vi "HandleObservationSync_002.vi"(8 "error in (no error)":errorcluster, 11 "S4GUI in":refnum<class "S4GUI.lvclass">) -> (0 "error out":errorcluster, 3 "S4GUI out":refnum<class "S4GUI.lvclass">)   [LabVIEW 2018, in "S4GUI.lvclass"] (continued)
            tunnel: [w1984 w1997] -> w1912
            tunnel: [w1983 w1996] -> w1911
            tunnel: [0 ("State") w1986] -> w1887
            frame False {
            }
            frame True {
              n759 = call-dynamic "Read Channel.vi"("error in (no error)"=w1999, "Acquisition in"=w2000) -> ("error out"=w1995:errorcluster, "Channel.lvclass"=w1994:refnum<class "Channel.lvclass">, "Acquisition out"=w1998:refnum<class "Acquisition.lvclass">)  [unwired: 7 in]
              n760 = call-dynamic "Read State Machine.vi"("error in (no error)"=w1995, "Device in"=w1994) -> ("error out"=w1988:errorcluster, "State Machine.lvclass"=w1990:refnum<class "State Machine.lvclass">, "Device out"=w1992:refnum<class "Channel.lvclass">)  [unwired: 7 in]
              n761 = call-dynamic "Read State.vi"("error in (no error)"=w1988, "State Machine in"=w1990) -> ("error out"=w1987:errorcluster, "State"=w1986:i32, "State Machine out"=w1989:refnum<class "State Machine.lvclass">)  [unwired: 7 in]
              n762 = call-dynamic "Write State Machine.vi"("error in (no error)"=w1987, "State Machine.lvclass"=w1989, "Device in"=w1992) -> ("error out"=w1991:errorcluster, "Device out"=w1993:refnum<class "Channel.lvclass">)  [unwired: 7 in]
              n763 = call-dynamic "Write Channel.vi"("error in (no error)"=w1991, "Channel.lvclass"=w1993, "Acquisition in"=w1998) -> ("error out"=w1996:errorcluster, "Acquisition out"=w1997:refnum<class "Acquisition.lvclass">)  [unwired: 7 in]
            }
          }
          n764 = call-dynamic "Write AcquisitionC.vi"("error in (no error)"=w1911, "Acquisition.lvclass"=w1912, "S4ACS_GUI in"=w1941) -> ("error out"=w1935:errorcluster, "S4ACS_GUI out"=w1934:refnum<class "S4GUI.lvclass">)  [unwired: 7 in]
          n765 = call-dynamic "Read AcquisitionD.vi"("error in (no error)"=w1935, "S4ACS_GUI in"=w1934) -> ("error out"=w1908:errorcluster, "Acquisition.lvclass"=w1910:refnum<class "Acquisition.lvclass">, "S4ACS_GUI out"=w1940:refnum<class "S4GUI.lvclass">)  [unwired: 7 in]
          n766 = call "Read connection.vi"("error in (no error)"=w1908, "Server in"=w1910) -> ("error out"=w1907:errorcluster, "connection"=w1906:bool, "Server out"=w1909:refnum<class "Acquisition.lvclass">)  [unwired: 7 in]
          n767 = case shown="True" w1906 {
            tunnel: w1909 -> [w1966 w1982]
            tunnel: w1907 -> [w1965 w1981]
            tunnel: [w1966 w1979] -> w1905
            tunnel: [w1965 w1978] -> w1904
            tunnel: [0 ("State") w1968] -> w1886
            frame False {
            }
            frame True {
              n768 = call-dynamic "Read Channel.vi"("error in (no error)"=w1981, "Acquisition in"=w1982) -> ("error out"=w1977:errorcluster, "Channel.lvclass"=w1976:refnum<class "Channel.lvclass">, "Acquisition out"=w1980:refnum<class "Acquisition.lvclass">)  [unwired: 7 in]
              n769 = call-dynamic "Read State Machine.vi"("error in (no error)"=w1977, "Device in"=w1976) -> ("error out"=w1970:errorcluster, "State Machine.lvclass"=w1972:refnum<class "State Machine.lvclass">, "Device out"=w1974:refnum<class "Channel.lvclass">)  [unwired: 7 in]
              n770 = call-dynamic "Read State.vi"("error in (no error)"=w1970, "State Machine in"=w1972) -> ("error out"=w1969:errorcluster, "State"=w1968:i32, "State Machine out"=w1971:refnum<class "State Machine.lvclass">)  [unwired: 7 in]
              n771 = call-dynamic "Write State Machine.vi"("error in (no error)"=w1969, "State Machine.lvclass"=w1971, "Device in"=w1974) -> ("error out"=w1973:errorcluster, "Device out"=w1975:refnum<class "Channel.lvclass">)  [unwired: 7 in]
              n772 = call-dynamic "Write Channel.vi"("error in (no error)"=w1973, "Channel.lvclass"=w1975, "Acquisition in"=w1980) -> ("error out"=w1978:errorcluster, "Acquisition out"=w1979:refnum<class "Acquisition.lvclass">)  [unwired: 7 in]
            }
          }
          n773 = call-dynamic "Write AcquisitionD.vi"("error in (no error)"=w1904, "Acquisition.lvclass"=w1905, "S4ACS_GUI in"=w1940) -> ("error out"=w1933:errorcluster, "S4ACS_GUI out"=w1898:refnum<class "S4GUI.lvclass">)  [unwired: 7 in]
          n774 = Equal?(x=w1890, y=w1889) -> (x = y?=w1894:bool)
          n775 = Equal?(x=w1899, y=w1889) -> (x = y?=w1903:bool)
          n776 = Equal?(x=w1890, y=w1888) -> (x = y?=w1893:bool)
          n777 = Equal?(x=w1899, y=w1888) -> (x = y?=w1902:bool)
          n778 = Equal?(x=w1890, y=w1887) -> (x = y?=w1892:bool)
          n779 = Equal?(x=w1899, y=w1887) -> (x = y?=w1901:bool)
          n780 = Equal?(x=w1890, y=w1886) -> (x = y?=w1891:bool)
          n781 = Equal?(x=w1899, y=w1886) -> (x = y?=w1900:bool)
          n782 = Compound Arithmetic op=ADD(w1889, w1888, w1887, w1886) -> (w1897:i32)
          n783 = Compound Arithmetic op=OR(w1894, w1893, w1892, w1891) -> (w1884:bool)
          n784 = Compound Arithmetic op=OR(w1903, w1902, w1901, w1900) -> (w1885:bool)
          n785 = Build Array(w1885, w1884) -> (w1883:bool[])
          n786 = Boolean Array To Number(Boolean array=w1883) -> (number=w1882:u32)
          n787 = case shown="0, Default" w1882 {
            tunnel: w1898 -> [w1948 w1956 w1960 w1964]
            tunnel: [w1947 w1955 w1959 w1963] -> w1895
            tunnel: w1897 -> [w1952 _ _ _]
            tunnel: w1896 -> [w1949 _ _ _]
            frame 0, Default {
              n788 = Equal To 0?(x=w1952) -> (x = 0?=w1951:bool)
              n789 = Select(t=u32 360, s=w1951, f=w1949) -> (s? t:f=w1946:u32)
              n790 = Bundle By Name(cluster=w1948, "Obs_state"=w1946) -> (w1947:refnum<class "S4GUI.lvclass">)
            }
            frame 1 {
              n791 = Bundle By Name(cluster=w1956, "Obs_state"=u32 1, "Error Msg"="ERROR: Some channel initialization failed. S4GUI:HandleObservationSync.vi state 272.") -> (w1955:refnum<class "S4GUI.lvclass">)
            }
            frame 2 {
              n792 = Bundle By Name(cluster=w1960, "Obs_state"=u32 1, "Error Msg"="ERROR: Some channel with invalid Exposition Time. S4GUI:HandleObservationSync.vi state 272.") -> (w1959:refnum<class "S4GUI.lvclass">)
            }
            frame 3 {
              n793 = Bundle By Name(cluster=w1964, "Obs_state"=u32 1, "Error Msg"="ERROR: Invalid configuration in the channels. S4GUI:HandleObservationSync.vi state 272.") -> (w1963:refnum<class "S4GUI.lvclass">)
            }
          }
        }
        frame 299 {
          # "Verifcando iniciação dos CICLO:"
          # "T= todos os canais ativos estão zerados."
          # "Exemplo de erro em \"Cycles_done\":\nchA; cycles_done=0; CCD_STATUS=ACTIVE;                                           Seqs_done=15;\nchA; cycles_done=0; CCD_STATUS=IDLE;                                                Seqs_done=16;   =>mudança de seq. com mesmo ciclo\nchA; cycles_done=1; CCD_STATUS=WAITING_EXPOSE_COMMAND; Seqs_done=0;\n\nchB; cycles_done=0; CCD_STATUS=ACTIVE;                                           Seqs_done=15;\nchB; cycles_done=1; CCD_STATUS=WAITING_EXPOSE_COMMAND; Seqs_done=0;     => mudança de seq com novo ciclo"
          # "T=canais receberam STOP"
          # "T= Todos os canais ativos no mesmo ciclo;\nF= Canais em ciclo diferente."
          # "Todos os CYCLES_DONE \nestão zerados?\nSe sim, vai para 327."
          # "Exemplo:\nSET #CYCLES 3\nSET #SEQ 4\ntotal de sequencias: 3 x 4 = 12\n\nseq.        CYCLES_DONE           SEQS_DONE\n1a.                     0                                 0\n2a.                     0                                 1 \n3a.                     0                                 2 \n4a.                     0                                 3 \n                          1                                 4\n5a.                     1                                 0 \n6a.                     1                                 1 \n7a.                     1                                 2 \n8a.                     1                                 3 \n                          2                                 4\n9a.                     2                                 0 \n10a.                   2                                 1 \n11a.                   2                                 2 \n12a.                   2                                 3 \n\nfim                    3                                 4"
          n794 = call-dynamic "Read AcquisitionA.vi"("error in (no error)"=w2089, "S4ACS_GUI in"=w2055) -> ("error out"=w2070:errorcluster, "Acquisition.lvclass"=w2071:refnum<class "Acquisition.lvclass">, "S4ACS_GUI out"=w2091:refnum<class "S4GUI.lvclass">)  [unwired: 7 in]
          n795 = call-dynamic "Read enabled.vi"("error in (no error)"=w2070, "Server in"=w2071) -> ("error out"=w2069:errorcluster, "enabled"=w2050:bool, "Server out"=w2068:refnum<class "Acquisition.lvclass">)  [unwired: 7 in]
          n796 = case shown="True" w2050 {
            tunnel: w2069 -> [w2181 w2197]
            tunnel: [w2182 w2195] -> w2092
            tunnel: [w2181 w2194] -> w2090
            tunnel: [u32 0 ("SequesDone") w2193] -> _
            tunnel: w2068 -> [w2182 w2192]
            tunnel: [TRUE w2191] -> w2054
            tunnel: [FALSE ("stopping") w2184] -> w2046
            frame False {
            }
            frame True {
              # "CYCLES_DONE = 0 ?"
              n797 = call-dynamic "Read Channel.vi"("error in (no error)"=w2197, "Acquisition in"=w2192) -> ("error out"=w2189:errorcluster, "Channel.lvclass"=w2190:refnum<class "Channel.lvclass">, "Acquisition out"=w2196:refnum<class "Acquisition.lvclass">)  [unwired: 7 in]
              n798 = call-dynamic "Read CyclesDone.vi"("error in (no error)"=w2189, "Channel in"=w2190) -> ("error out"=w2187:errorcluster, "CyclesDone"=w2193:u32, "Channel out"=w2188:refnum<class "Channel.lvclass">)  [unwired: 7 in]
              n799 = Equal?(x=w2193, y=u32 0) -> (x = y?=w2191:bool)
              n800 = call-dynamic "Read stopping.vi"("error in (no error)"=w2187, "Channel in"=w2188) -> ("error out"=w2186:errorcluster, "stopping"=w2184:bool, "Channel out"=w2185:refnum<class "Channel.lvclass">)  [unwired: 7 in]
              n801 = call-dynamic "Write Channel.vi"("error in (no error)"=w2186, "Channel.lvclass"=w2185, "Acquisition in"=w2196) -> ("error out"=w2194:errorcluster, "Acquisition out"=w2195:refnum<class "Acquisition.lvclass">)  [unwired: 7 in]
            }
          }
          n802 = call-dynamic "Write AcquisitionA.vi"("error in (no error)"=w2090, "Acquisition.lvclass"=w2092, "S4ACS_GUI in"=w2091) -> ("error out"=w2087:errorcluster, "S4ACS_GUI out"=w2086:refnum<class "S4GUI.lvclass">)  [unwired: 7 in]
          n803 = call "Read AcquisitionB.vi"("error in (no error)"=w2087, "S4ACS_GUI in"=w2086) -> ("error out"=w2064:errorcluster, "Acquisition.lvclass"=w2067:refnum<class "Acquisition.lvclass">, "S4ACS_GUI out"=w2088:refnum<class "S4GUI.lvclass">)  [unwired: 7 in]
          n804 = call-dynamic "Read enabled.vi"("error in (no error)"=w2064, "Server in"=w2067) -> ("error out"=w2065:errorcluster, "enabled"=w2049:bool, "Server out"=w2066:refnum<class "Acquisition.lvclass">)  [unwired: 7 in]
          n805 = case shown="True" w2049 {
            tunnel: w2065 -> [w2161 w2177]
            tunnel: w2066 -> [w2162 w2176]
            tunnel: [u32 0 ("SequesDone") w2171] -> _
            tunnel: [w2161 w2175] -> w2085
            tunnel: [w2162 w2174] -> w2084
            tunnel: [TRUE w2170] -> w2053
            tunnel: [FALSE ("stopping") w2164] -> w2045
            frame False {
            }
            frame True {
              n806 = call-dynamic "Read Channel.vi"("error in (no error)"=w2177, "Acquisition in"=w2176) -> ("error out"=w2168:errorcluster, "Channel.lvclass"=w2169:refnum<class "Channel.lvclass">, "Acquisition out"=w2172:refnum<class "Acquisition.lvclass">)  [unwired: 7 in]
              n807 = call-dynamic "Read CyclesDone.vi"("error in (no error)"=w2168, "Channel in"=w2169) -> ("error out"=w2166:errorcluster, "CyclesDone"=w2171:u32, "Channel out"=w2173:refnum<class "Channel.lvclass">)  [unwired: 7 in]
              n808 = Equal?(x=w2171, y=u32 0) -> (x = y?=w2170:bool)
              n809 = call-dynamic "Read stopping.vi"("error in (no error)"=w2166, "Channel in"=w2173) -> ("error out"=w2165:errorcluster, "stopping"=w2164:bool, "Channel out"=w2167:refnum<class "Channel.lvclass">)  [unwired: 7 in]
              n810 = call-dynamic "Write Channel.vi"("error in (no error)"=w2165, "Channel.lvclass"=w2167, "Acquisition in"=w2172) -> ("error out"=w2175:errorcluster, "Acquisition out"=w2174:refnum<class "Acquisition.lvclass">)  [unwired: 7 in]
            }
          }
          n811 = call "Write AcquisitionB.vi"("error in (no error)"=w2085, "Acquisition.lvclass"=w2084, "S4ACS_GUI in"=w2088) -> ("error out"=w2077:errorcluster, "S4ACS_GUI out"=w2076:refnum<class "S4GUI.lvclass">)  [unwired: 7 in]
          n812 = call-dynamic "Read AcquisitionC.vi"("error in (no error)"=w2077, "S4ACS_GUI in"=w2076) -> ("error out"=w2061:errorcluster, "Acquisition.lvclass"=w2063:refnum<class "Acquisition.lvclass">, "S4ACS_GUI out"=w2079:refnum<class "S4GUI.lvclass">)  [unwired: 7 in]
          n813 = call-dynamic "Read enabled.vi"("error in (no error)"=w2061, "Server in"=w2063) -> ("error out"=w2060:errorcluster, "enabled"=w2048:bool, "Server out"=w2062:refnum<class "Acquisition.lvclass">)  [unwired: 7 in]
          n814 = case shown="True" w2048 {
            tunnel: [w2141 w2157] -> w2080
            tunnel: [w2142 w2156] -> w2078
            tunnel: w2060 -> [w2141 w2153]
            tunnel: w2062 -> [w2142 w2154]
            tunnel: [u32 0 ("SequesDone") w2152] -> _
            tunnel: [TRUE w2151] -> w2052
            tunnel: [FALSE ("stopping") w2144] -> w2044
            frame False {
            }
            frame True {
              n815 = call-dynamic "Read Channel.vi"("error in (no error)"=w2153, "Acquisition in"=w2154) -> ("error out"=w2148:errorcluster, "Channel.lvclass"=w2149:refnum<class "Channel.lvclass">, "Acquisition out"=w2155:refnum<class "Acquisition.lvclass">)  [unwired: 7 in]
              n816 = call-dynamic "Read CyclesDone.vi"("error in (no error)"=w2148, "Channel in"=w2149) -> ("error out"=w2146:errorcluster, "CyclesDone"=w2152:u32, "Channel out"=w2150:refnum<class "Channel.lvclass">)  [unwired: 7 in]
              n817 = Equal?(x=w2152, y=u32 0) -> (x = y?=w2151:bool)
              n818 = call-dynamic "Read stopping.vi"("error in (no error)"=w2146, "Channel in"=w2150) -> ("error out"=w2145:errorcluster, "stopping"=w2144:bool, "Channel out"=w2147:refnum<class "Channel.lvclass">)  [unwired: 7 in]
              n819 = call-dynamic "Write Channel.vi"("error in (no error)"=w2145, "Channel.lvclass"=w2147, "Acquisition in"=w2155) -> ("error out"=w2157:errorcluster, "Acquisition out"=w2156:refnum<class "Acquisition.lvclass">)  [unwired: 7 in]
            }
          }
          n820 = call-dynamic "Write AcquisitionC.vi"("error in (no error)"=w2080, "Acquisition.lvclass"=w2078, "S4ACS_GUI in"=w2079) -> ("error out"=w2074:errorcluster, "S4ACS_GUI out"=w2075:refnum<class "S4GUI.lvclass">)  [unwired: 7 in]
          n821 = call-dynamic "Read AcquisitionD.vi"("error in (no error)"=w2074, "S4ACS_GUI in"=w2075) -> ("error out"=w2057:errorcluster, "Acquisition.lvclass"=w2059:refnum<class "Acquisition.lvclass">, "S4ACS_GUI out"=w2081:refnum<class "S4GUI.lvclass">)  [unwired: 7 in]
          n822 = call-dynamic "Read enabled.vi"("error in (no error)"=w2057, "Server in"=w2059) -> ("error out"=w2056:errorcluster, "enabled"=w2047:bool, "Server out"=w2058:refnum<class "Acquisition.lvclass">)  [unwired: 7 in]
          n823 = case shown="True" w2047 {
            tunnel: [w2122 w2137] -> w2083
            tunnel: [w2121 w2136] -> w2082
            tunnel: w2058 -> [w2122 w2135]
            tunnel: w2056 -> [w2121 w2134]
            tunnel: [u32 0 ("SequesDone") w2132] -> _
            tunnel: [TRUE w2131] -> w2051
            tunnel: [FALSE ("stopping") w2124] -> w2043
            frame False {
            }
            frame True {
              n824 = call-dynamic "Read Channel.vi"("error in (no error)"=w2134, "Acquisition in"=w2135) -> ("error out"=w2128:errorcluster, "Channel.lvclass"=w2129:refnum<class "Channel.lvclass">, "Acquisition out"=w2133:refnum<class "Acquisition.lvclass">)  [unwired: 7 in]
              n825 = call-dynamic "Read CyclesDone.vi"("error in (no error)"=w2128, "Channel in"=w2129) -> ("error out"=w2126:errorcluster, "CyclesDone"=w2132:u32, "Channel out"=w2130:refnum<class "Channel.lvclass">)  [unwired: 7 in]
              n826 = Equal?(x=w2132, y=u32 0) -> (x = y?=w2131:bool)
              n827 = call-dynamic "Read stopping.vi"("error in (no error)"=w2126, "Channel in"=w2130) -> ("error out"=w2125:errorcluster, "stopping"=w2124:bool, "Channel out"=w2127:refnum<class "Channel.lvclass">)  [unwired: 7 in]
              n828 = call-dynamic "Write Channel.vi"("error in (no error)"=w2125, "Channel.lvclass"=w2127, "Acquisition in"=w2133) -> ("error out"=w2136:errorcluster, "Acquisition out"=w2137:refnum<class "Acquisition.lvclass">)  [unwired: 7 in]
            }
          }
          n829 = Compound Arithmetic op=AND(w2054, w2053, w2052, w2051) -> (w2040:bool)
          n830 = Compound Arithmetic op=OR(w2046, w2045, w2044, w2043) -> (w2042:bool)
          n831 = call-dynamic "Write AcquisitionD.vi"("error in (no error)"=w2082, "Acquisition.lvclass"=w2083, "S4ACS_GUI in"=w2081) -> ("error out"=w2072:errorcluster, "S4ACS_GUI out"=w2073:refnum<class "S4GUI.lvclass">)  [unwired: 7 in]
          n832 = case shown="True" w2040 {
            tunnel: w2073 -> [w2103 w2114]
            tunnel: [w2102 w2113] -> w2041
            tunnel: w2042 -> [_ w2112]
            tunnel: w2039 -> [_ w2109]
            frame False {
              # "Esperando todos os canais habilitados mudarem de cyclesDone.\nE verificando a maior duracao de cubo entre os canais."
              n833 = local read "time307"() -> (w2101:u32)
              n834 = Tick Count (ms)() -> (millisecond timer value=w2100:u32)
              n835 = Subtract(x=w2100, y=w2101) -> (x-y=w2096:u32)
              n836 = call-dynamic "GetGreatestCube.vi"("S4GUI in"=w2103) -> ("S4GUI out"=w2098:refnum<class "S4GUI.lvclass">, "greatest (ms)"=w2094:dbl)  [unwired: 8 in, 1 out]
              n837 = To Double Precision Float(number=w2096) -> (double precision float=w2099:dbl)
              n838 = Add(x=1000.0 ("y"), y=w2094) -> (x+y=w2093:dbl)
              n839 = Less?(x=w2093, y=w2099) -> (x < y?=w2097:bool)
              n840 = case shown="True" w2097 {
                tunnel: w2098 -> [w2104 w2108]
                tunnel: [w2104 w2107] -> w2102
                frame False {
                }
                frame True {
                  n841 = Bundle By Name(cluster=w2108, "Obs_state"=u32 1, "Error Msg"="ERROR: Cycles_Done reseting timeout. - HandleObservationSync.vi state 299.") -> (w2107:refnum<class "S4GUI.lvclass">)
                }
              }
            }
            frame True {
              # "STOP?"
              n842 = case shown="False" w2112 {
                tunnel: [w2115 u32 0] -> w2111
                tunnel: w2109 -> [w2116 _]
                frame False {
                  n843 = Increment(x=w2116) -> (x+1=w2115:u32)
                }
                frame True {
                }
              }
              n844 = Bundle By Name(cluster=w2114, "Obs_state"=w2111, "cyclesDone"=u32 0) -> (w2113:refnum<class "S4GUI.lvclass">)
            }
          }
        }
        frame 300 {
          # "Verifica se é modo fotometria ou polarimetria:\nTrue = polarimetria (esatdo 301)\nFalse = fotometria (estado 321)"
          n845 = flat-sequence {
            tunnel: w2202 -> [w2215]
            tunnel: [w2215] -> w2201
            frame #0 {
              n846 = local read "time3"() -> (w2217:u32)
              n847 = local read "time4"() -> (w2214:u32)
              n848 = Tick Count (ms)() -> (millisecond timer value=w2213:u32)
              n849 = Subtract(x=w2214, y=w2217) -> (x-y=→"delay 3-4":u32)
              n850 = local write "time1"(w2213) -> ()
            }
          }
          n851 = call "Read Instrument.lvclass.vi"("error in (no error)"=w2201, "S4ACS_GUI in"=w2212) -> ("error out"=w2207:errorcluster, "Instrument.lvclass"=w2208:refnum<class "Instrument.lvclass">, "S4ACS_GUI out"=w2206:refnum<class "S4GUI.lvclass">)  [unwired: 7 in]
          n852 = call-dynamic "Read mode.vi"("error in (no error)"=w2207, "Instrument in"=w2208) -> ("error out"=w2203:errorcluster, "mode"=w2205:bool)  [unwired: 7 in, 1 out]
          n853 = Select(t=u32 301, s=w2205, f=u32 321 ("t")) -> (s? t:f=w2210:u32)
          n854 = Bundle By Name(cluster=w2206, "Obs_state"=w2210, "cyclesDone"=u32 0, "sequesDone"=u32 0, "seqAtual"=u32 0) -> (w2211:refnum<class "S4GUI.lvclass">)
        }
        frame 301 {
          # "Configurando para ACS esperar comando EXPOSE"
          n855 = call-dynamic "Read AcquisitionA.vi"("error in (no error)"=w2280, "S4ACS_GUI in"=w2281) -> ("error out"=w2235:errorcluster, "Acquisition.lvclass"=w2236:refnum<class "Acquisition.lvclass">, "S4ACS_GUI out"=w2283:refnum<class "S4GUI.lvclass">)  [unwired: 7 in]
          n856 = call-dynamic "Read enabled.vi"("error in (no error)"=w2235, "Server in"=w2236) -> ("error out"=w2234:errorcluster, "enabled"=w2221:bool, "Server out"=w2237:refnum<class "Acquisition.lvclass">)  [unwired: 7 in]
          n857 = call "Read connection.vi"("error in (no error)"=w2234, "Server in"=w2237) -> ("error out"=w2260:errorcluster, "connection"=w2244:bool, "Server out"=w2261:refnum<class "Acquisition.lvclass">)  [unwired: 7 in]
          n858 = And(x=w2244, y=w2221) -> (x .and. y?=w2245:bool)
          n859 = case shown="True" w2245 {
            tunnel: w2261 -> [w2398 w2417]
            tunnel: w2260 -> [w2397 w2416]
            tunnel: [w2398 w2414] -> w2284
            tunnel: [w2397 w2413] -> w2282
            tunnel: [w2394 u32 0 ("New_State")] -> w2250
            tunnel: w2221 -> [w2393 _]
            frame False {
              n860 = Select(t=u32 1, s=w2393, f=u32 0) -> (s? t:f=w2394:u32)
            }
            frame True {
              n861 = call-dynamic "Read Channel.vi"("error in (no error)"=w2416, "Acquisition in"=w2417) -> ("error out"=w2400:errorcluster, "Channel.lvclass"=w2403:refnum<class "Channel.lvclass">, "Acquisition out"=w2415:refnum<class "Acquisition.lvclass">)  [unwired: 7 in]
              n862 = call-dynamic "Write wait_expose.vi"("error in (no error)"=w2400, "wait_expose"=TRUE, "Channel in"=w2403) -> ("error out"=w2399:errorcluster, "Channel out"=w2402:refnum<class "Channel.lvclass">)  [unwired: 7 in]
              n863 = call-dynamic "Read State Machine.vi"("error in (no error)"=w2399, "Device in"=w2402) -> ("error out"=w2410:errorcluster, "State Machine.lvclass"=w2412:refnum<class "State Machine.lvclass">, "Device out"=w2408:refnum<class "Channel.lvclass">)  [unwired: 7 in]
              n864 = call "Next State.vi"("error in (no error)"=w2410, "New_State"=40, "State Machine in"=w2412) -> ("error out"=w2405:errorcluster, "State Machine out"=w2406:refnum<class "State Machine.lvclass">)  [unwired: 7 in]
              n865 = call-dynamic "Write State Machine.vi"("error in (no error)"=w2405, "State Machine.lvclass"=w2406, "Device in"=w2408) -> ("error out"=w2407:errorcluster, "Device out"=w2409:refnum<class "Channel.lvclass">)  [unwired: 7 in]
              n866 = call-dynamic "Write Channel.vi"("error in (no error)"=w2407, "Channel.lvclass"=w2409, "Acquisition in"=w2415) -> ("error out"=w2413:errorcluster, "Acquisition out"=w2414:refnum<class "Acquisition.lvclass">)  [unwired: 7 in]
            }
          }
          n867 = call-dynamic "Write AcquisitionA.vi"("error in (no error)"=w2282, "Acquisition.lvclass"=w2284, "S4ACS_GUI in"=w2283) -> ("error out"=w2277:errorcluster, "S4ACS_GUI out"=w2278:refnum<class "S4GUI.lvclass">)  [unwired: 7 in]
          n868 = call "Read AcquisitionB.vi"("error in (no error)"=w2277, "S4ACS_GUI in"=w2278) -> ("error out"=w2231:errorcluster, "Acquisition.lvclass"=w2233:refnum<class "Acquisition.lvclass">, "S4ACS_GUI out"=w2275:refnum<class "S4GUI.lvclass">)  [unwired: 7 in]
          n869 = call-dynamic "Read enabled.vi"("error in (no error)"=w2231, "Server in"=w2233) -> ("error out"=w2230:errorcluster, "enabled"=w2220:bool, "Server out"=w2232:refnum<class "Acquisition.lvclass">)  [unwired: 7 in]
          n870 = call "Read connection.vi"("error in (no error)"=w2230, "Server in"=w2232) -> ("error out"=w2258:errorcluster, "connection"=w2242:bool, "Server out"=w2259:refnum<class "Acquisition.lvclass">)  [unwired: 7 in]
          n871 = And(x=w2242, y=w2220) -> (x .and. y?=w2243:bool)
          n872 = case shown="True" w2243 {
            tunnel: w2259 -> [w2373 w2392]
            tunnel: w2258 -> [w2372 w2391]
            tunnel: [w2373 w2389] -> w2276
            tunnel: [w2372 w2388] -> w2274
            tunnel: [w2369 u32 0 ("New_State")] -> w2249
            tunnel: w2220 -> [w2368 _]
            frame False {
              n873 = Select(t=u32 2, s=w2368, f=u32 0) -> (s? t:f=w2369:u32)
            }
            frame True {
              n874 = call-dynamic "Read Channel.vi"("error in (no error)"=w2391, "Acquisition in"=w2392) -> ("error out"=w2375:errorcluster, "Channel.lvclass"=w2377:refnum<class "Channel.lvclass">, "Acquisition out"=w2390:refnum<class "Acquisition.lvclass">)  [unwired: 7 in]
              n875 = call-dynamic "Write wait_expose.vi"("error in (no error)"=w2375, "wait_expose"=TRUE, "Channel in"=w2377) -> ("error out"=w2374:errorcluster, "Channel out"=w2376:refnum<class "Channel.lvclass">)  [unwired: 7 in]
              n876 = call-dynamic "Read State Machine.vi"("error in (no error)"=w2374, "Device in"=w2376) -> ("error out"=w2385:errorcluster, "State Machine.lvclass"=w2387:refnum<class "State Machine.lvclass">, "Device out"=w2383:refnum<class "Channel.lvclass">)  [unwired: 7 in]
              n877 = call "Next State.vi"("error in (no error)"=w2385, "New_State"=40, "State Machine in"=w2387) -> ("error out"=w2380:errorcluster, "State Machine out"=w2381:refnum<class "State Machine.lvclass">)  [unwired: 7 in]
              n878 = call-dynamic "Write State Machine.vi"("error in (no error)"=w2380, "State Machine.lvclass"=w2381, "Device in"=w2383) -> ("error out"=w2382:errorcluster, "Device out"=w2384:refnum<class "Channel.lvclass">)  [unwired: 7 in]
              n879 = call-dynamic "Write Channel.vi"("error in (no error)"=w2382, "Channel.lvclass"=w2384, "Acquisition in"=w2390) -> ("error out"=w2388:errorcluster, "Acquisition out"=w2389:refnum<class "Acquisition.lvclass">)  [unwired: 7 in]
            }
          }
          n880 = call "Write AcquisitionB.vi"("error in (no error)"=w2274, "Acquisition.lvclass"=w2276, "S4ACS_GUI in"=w2275) -> ("error out"=w2270:errorcluster, "S4ACS_GUI out"=w2269:refnum<class "S4GUI.lvclass">)  [unwired: 7 in]
          n881 = call-dynamic "Read AcquisitionC.vi"("error in (no error)"=w2270, "S4ACS_GUI in"=w2269) -> ("error out"=w2227:errorcluster, "Acquisition.lvclass"=w2229:refnum<class "Acquisition.lvclass">, "S4ACS_GUI out"=w2272:refnum<class "S4GUI.lvclass">)  [unwired: 7 in]
          n882 = call-dynamic "Read enabled.vi"("error in (no error)"=w2227, "Server in"=w2229) -> ("error out"=w2226:errorcluster, "enabled"=w2219:bool, "Server out"=w2228:refnum<class "Acquisition.lvclass">)  [unwired: 7 in]
          n883 = call "Read connection.vi"("error in (no error)"=w2226, "Server in"=w2228) -> ("error out"=w2256:errorcluster, "connection"=w2239:bool, "Server out"=w2257:refnum<class "Acquisition.lvclass">)  [unwired: 7 in]
          n884 = And(x=w2239, y=w2219) -> (x .and. y?=w2241:bool)
          n885 = case shown="True" w2241 {
            tunnel: [w2347 w2361] -> w2273
            tunnel: [w2348 w2360] -> w2271
            tunnel: w2257 -> [w2348 w2358]
            tunnel: w2256 -> [w2347 w2357]
            tunnel: [w2344 u32 0 ("New_State")] -> w2248
            tunnel: w2219 -> [w2343 _]
            frame False {
              n886 = Select(t=u32 4, s=w2343, f=u32 0) -> (s? t:f=w2344:u32)
            }
            frame True {
              n887 = call-dynamic "Read Channel.vi"("error in (no error)"=w2357, "Acquisition in"=w2358) -> ("error out"=w2350:errorcluster, "Channel.lvclass"=w2352:refnum<class "Channel.lvclass">, "Acquisition out"=w2359:refnum<class "Acquisition.lvclass">)  [unwired: 7 in]
              n888 = call-dynamic "Write wait_expose.vi"("error in (no error)"=w2350, "wait_expose"=TRUE, "Channel in"=w2352) -> ("error out"=w2349:errorcluster, "Channel out"=w2351:refnum<class "Channel.lvclass">)  [unwired: 7 in]
              n889 = call-dynamic "Read State Machine.vi"("error in (no error)"=w2349, "Device in"=w2351) -> ("error out"=w2364:errorcluster, "State Machine.lvclass"=w2362:refnum<class "State Machine.lvclass">, "Device out"=w2366:refnum<class "Channel.lvclass">)  [unwired: 7 in]
              n890 = call "Next State.vi"("error in (no error)"=w2364, "New_State"=40, "State Machine in"=w2362) -> ("error out"=w2356:errorcluster, "State Machine out"=w2355:refnum<class "State Machine.lvclass">)  [unwired: 7 in]
              n891 = call-dynamic "Write State Machine.vi"("error in (no error)"=w2356, "State Machine.lvclass"=w2355, "Device in"=w2366) -> ("error out"=w2367:errorcluster, "Device out"=w2365:refnum<class "Channel.lvclass">)  [unwired: 7 in]
              n892 = call-dynamic "Write Channel.vi"("error in (no error)"=w2367, "Channel.lvclass"=w2365, "Acquisition in"=w2359) -> ("error out"=w2361:errorcluster, "Acquisition out"=w2360:refnum<class "Acquisition.lvclass">)  [unwired: 7 in]
            }
          }
          n893 = call-dynamic "Write AcquisitionC.vi"("error in (no error)"=w2273, "Acquisition.lvclass"=w2271, "S4ACS_GUI in"=w2272) -> ("error out"=w2267:errorcluster, "S4ACS_GUI out"=w2266:refnum<class "S4GUI.lvclass">)  [unwired: 7 in]
          n894 = call-dynamic "Read AcquisitionD.vi"("error in (no error)"=w2267, "S4ACS_GUI in"=w2266) -> ("error out"=w2223:errorcluster, "Acquisition.lvclass"=w2225:refnum<class "Acquisition.lvclass">, "S4ACS_GUI out"=w2265:refnum<class "S4GUI.lvclass">)  [unwired: 7 in]
          n895 = call-dynamic "Read enabled.vi"("error in (no error)"=w2223, "Server in"=w2225) -> ("error out"=w2222:errorcluster, "enabled"=w2218:bool, "Server out"=w2224:refnum<class "Acquisition.lvclass">)  [unwired: 7 in]
          n896 = call "Read connection.vi"("error in (no error)"=w2222, "Server in"=w2224) -> ("error out"=w2254:errorcluster, "connection"=w2238:bool, "Server out"=w2255:refnum<class "Acquisition.lvclass">)  [unwired: 7 in]
          n897 = And(x=w2238, y=w2218) -> (x .and. y?=w2240:bool)
          n898 = case shown="True" w2240 {
            tunnel: w2254 -> [w2322 w2342]
            tunnel: [w2322 w2341] -> w2268
            tunnel: w2255 -> [w2323 w2334]
            tunnel: [w2323 w2332] -> w2264
            tunnel: [w2319 u32 0 ("New_State")] -> w2247
            tunnel: w2218 -> [w2318 _]
            frame False {
              n899 = Select(t=u32 8, s=w2318, f=u32 0) -> (s? t:f=w2319:u32)
            }
            frame True {
              n900 = call-dynamic "Read Channel.vi"("error in (no error)"=w2342, "Acquisition in"=w2334) -> ("error out"=w2324:errorcluster, "Channel.lvclass"=w2327:refnum<class "Channel.lvclass">, "Acquisition out"=w2333:refnum<class "Acquisition.lvclass">)  [unwired: 7 in]
              n901 = call-dynamic "Write wait_expose.vi"("error in (no error)"=w2324, "wait_expose"=TRUE, "Channel in"=w2327) -> ("error out"=w2325:errorcluster, "Channel out"=w2326:refnum<class "Channel.lvclass">)  [unwired: 7 in]
              n902 = call-dynamic "Read State Machine.vi"("error in (no error)"=w2325, "Device in"=w2326) -> ("error out"=w2338:errorcluster, "State Machine.lvclass"=w2340:refnum<class "State Machine.lvclass">, "Device out"=w2336:refnum<class "Channel.lvclass">)  [unwired: 7 in]
              n903 = call "Next State.vi"("error in (no error)"=w2338, "New_State"=40, "State Machine in"=w2340) -> ("error out"=w2330:errorcluster, "State Machine out"=w2331:refnum<class "State Machine.lvclass">)  [unwired: 7 in]
              n904 = call-dynamic "Write State Machine.vi"("error in (no error)"=w2330, "State Machine.lvclass"=w2331, "Device in"=w2336) -> ("error out"=w2335:errorcluster, "Device out"=w2337:refnum<class "Channel.lvclass">)  [unwired: 7 in]
              n905 = call-dynamic "Write Channel.vi"("error in (no error)"=w2335, "Channel.lvclass"=w2337, "Acquisition in"=w2333) -> ("error out"=w2341:errorcluster, "Acquisition out"=w2332:refnum<class "Acquisition.lvclass">)  [unwired: 7 in]
            }
          }
          n906 = call-dynamic "Write AcquisitionD.vi"("error in (no error)"=w2268, "Acquisition.lvclass"=w2264, "S4ACS_GUI in"=w2265) -> ("error out"=w2263:errorcluster, "S4ACS_GUI out"=w2262:refnum<class "S4GUI.lvclass">)  [unwired: 7 in]
          n907 = Compound Arithmetic op=ADD(w2250, w2249, w2248, w2247) -> (w2251:u32)
          n908 = case shown="0, Default" w2251 {
            tunnel: w2246 -> [w2287 _ _ _ _ _ _ _ _ _ _ _ _ _ _ _]
            tunnel: [w2286 u32 1 ("Obs_state") u32 1 ("Obs_state") u32 1 ("Obs_state") u32 1 ("Obs_state") u32 1 ("Obs_state") u32 1 ("Obs_state") u32 1 ("Obs_state") u32 1 ("Obs_state") u32 1 ("Obs_state") u32 1 ("Obs_state") u32 1 ("Obs_state") u32 1 ("Obs_state") u32 1 ("Obs_state") u32 1 ("Obs_state") u32 1 ("Obs_state")] -> w2252
            tunnel: ["" ("Error Msg") "ERROR: Lost channel 1 connection... - HandleObservationSync.vi state 301" ("Error Msg") "ERROR: Lost channel 2 connection...- HandleObservationSync.vi state 301" ("Error Msg") "ERROR: Lost channels 1 and 2 connection...- HandleObservationSync.vi state 301" ("Error Msg") "ERROR: Lost channel 3 connection...- HandleObservationSync.vi state 301" ("Error Msg") "ERROR: Lost channels 1 and  3 connection...- HandleObservationSync.vi state 301" ("Error Msg") "ERROR:  Lost channels 2 and  3 connection...- HandleObservationSync.vi state 301" ("Error Msg") "ERROR:  Lost channels 1, 2 and  3 connection...- HandleObservationSync.vi state 301" ("Error Msg") "ERROR: Lost channel 4 connection...- HandleObservationSync.vi state 301" ("Error Msg") "ERROR:  Lost channels 1 and 4 connection...- HandleObservationSync.vi state 301" ("Error Msg") "ERROR:  Lost channels 2 and 4 connection...- HandleObservationSync.vi state 301" ("Error Msg") "ERROR: Lost channels 1, 2 and 4 connection...- HandleObservationSync.vi state 301" ("Error Msg") "ERROR: Lost channels 3 and 4 connection...- HandleObservationSync.vi state 301" ("Error Msg") "ERROR: Lost channels 1, 3 and 4 connection...- HandleObservationSync.vi state 301" ("Error Msg") "ERROR: Lost channels 2, 3 and 4 connection...- HandleObservationSync.vi state 301" ("Error Msg") "ERROR: Lost channels 1, 2, 3 and 4 connection...- HandleObservationSync.vi state 301" ("Error Msg")] -> w2253
            frame 0, Default {
              n909 = Increment(x=w2287) -> (x+1=w2286:u32)
            }
            frame 1 {
            }
            frame 2 {
            }
            frame 3 {
            }
            frame 4 {
            }
            frame 5 {
            }
            frame 6 {
            }
            frame 7 {
            }
            frame 8 {
            }
            frame 9 {
            }
            frame 10 {
            }
            frame 11 {
            }
            frame 12 {
            }
            frame 13 {
            }
            frame 14 {
            }
            frame 15 {
            }
          }
          n910 = Bundle By Name(cluster=w2262, "Obs_state"=w2252, "Error Msg"=w2253) -> (w2279:refnum<class "S4GUI.lvclass">)
        }
        frame 302 {
          # "Espera terminar o envio de WAIT EXPOSE COMMAND para todos os ACS."
          n911 = call-dynamic "VerifyAcqIdle.vi"("error in (no error)"=w2419, "S4GUI in"=w2418) -> ("error out"=w2424:errorcluster, "idle"=w2423:bool, "S4GUI out"=w2425:refnum<class "S4GUI.lvclass">)  [unwired: 7 in]
          n912 = Increment(x=w2421) -> (x+1=w2420:u32)
          n913 = Select(t=w2420, s=w2423, f=w2421) -> (s? t:f=w2422:u32)
          n914 = Bundle By Name(cluster=w2425, "Obs_state"=w2422) -> (w2426:refnum<class "S4GUI.lvclass">)
        }
        frame 303 {
          n915 = flat-sequence {
            tunnel: w2432 -> [w2471]
            tunnel: [w2471] -> w2431
            frame #0 {
              n916 = Tick Count (ms)() -> (millisecond timer value=→"time1":u32)
            }
          }
          n917 = call "Read Instrument.lvclass.vi"("error in (no error)"=w2431, "S4ACS_GUI in"=w2467) -> ("error out"=w2469:errorcluster, "Instrument.lvclass"=w2470:refnum<class "Instrument.lvclass">, "S4ACS_GUI out"=w2428:refnum<class "S4GUI.lvclass">)  [unwired: 7 in]
          n918 = call "Read WPROT.vi"("error in (no error)"=w2469, "Instrument in"=w2470) -> ("error out"=w2460:errorcluster, "Opt_Selector.lvclass"=w2461:refnum<class "Opt_Selector.lvclass">, "Instrument out"=w2468:refnum<class "Instrument.lvclass">)  [unwired: 7 in]
          n919 = call-dynamic "getTargetPos.vi"("error in (no error)"=w2460, "Opt_Selector in"=w2461) -> ("error out"=w2459:errorcluster, "Target Pos"=w2439:u16, "Opt_Selector out"=w2458:refnum<class "Opt_Selector.lvclass">)  [unwired: 7 in]
          n920 = Build Array(-1.0 ("element"), 0.0 ("element"), 22.5 ("element"), 45.0 ("element"), 67.5 ("element"), 90.0 ("element"), 112.5 ("element"), 135.0 ("element"), 157.5 ("element"), 180.0 ("element"), 202.5 ("element"), 225.0 ("element"), 247.5 ("element"), 270.0 ("element"), 292.5 ("element"), 315.0 ("element"), 337.5 ("element")) -> (w2451:dbl[])
          n921 = Index Array(array=w2451, index=w2439) -> (element=w2438:dbl)
          n922 = Unbundle By Name(w2428) -> ("seqAtual"=w2430:u32)
          n923 = case shown="0, Default" w2439 {
            selector: w2439 -> [_ w2505]
            tunnel: w2468 -> [w2481 w2493]
            tunnel: [w2481 w2493] -> w2434
            tunnel: [w2478 w2492] -> w2433
            tunnel: w2464 -> [_ w2507]
            tunnel: [u32 314 w2506] -> w2463
            tunnel: w2459 -> [w2479 w2501]
            tunnel: w2458 -> [w2480 w2500]
            tunnel: w2438 -> [_ w2495]
            tunnel: [w2476 w2494] -> w2435
            tunnel: [u32 0 w2483] -> w2429
            tunnel: w2430 -> [_ w2484]
            frame 0, Default {
              # "Terminou uma sequência.\nRecupera as posições em SEQ e desvia para 314 para verificar se há mais ciclos."
              # "Recupera a sequencia anterior para o caso \nde repetição da sequencia (sem precisar clicar \nnas posicoes desejadas novamente)."
              n924 = call-dynamic "Read sequencia_ant.vi"("error in (no error)"=w2479, "Opt_Selector in"=w2480) -> ("error out"=w2475:errorcluster, "sequencia_ant"=w2474:u16, "Opt_Selector out"=w2477:refnum<class "Opt_Selector.lvclass">)  [unwired: 7 in]
              n925 = call-dynamic "Write sequencia.vi"("error in (no error)"=w2475, "sequencia"=w2474, "Opt_Selector in"=w2477) -> ("error out"=w2478:errorcluster, "Opt_Selector out"=w2476:refnum<class "Opt_Selector.lvclass">)  [unwired: 7 in]
            }
            frame 1..16 {
              # "Inicia o Ticks com\nvalor do relogio atual"
              # "Espera até 40 x 0.25s (= 10s) para\nmecanismo entrar em READY"
              n926 = Number To Decimal String(number=w2505) -> (decimal integer string=w2504:string)  [unwired: 1 in]
              n927 = Concatenate Strings("WP" ("string"), w2504) -> (w2502:string)
              n928 = call "Write target name.vi"("error in (no error)"=w2501, "target name"=w2502, "Optics in"=w2500) -> ("error out"=w2498:errorcluster, "Optics out"=w2499:refnum<class "Opt_Selector.lvclass">)  [unwired: 7 in]
              n929 = call "Write target.vi"("error in (no error)"=w2498, "target"=w2495, "Optics in"=w2499) -> ("error out"=w2497:errorcluster, "Optics out"=w2496:refnum<class "Opt_Selector.lvclass">)  [unwired: 7 in]
              n930 = call-dynamic "Read State Machine.vi"("error in (no error)"=w2497, "Device in"=w2496) -> ("error out"=w2509:errorcluster, "State Machine.lvclass"=w2511:refnum<class "State Machine.lvclass">, "Device out"=w2508:refnum<class "Opt_Selector.lvclass">)  [unwired: 7 in]
              n931 = Increment(x=w2507) -> (x+1=w2506:u32)
              n932 = call "Next State.vi"("error in (no error)"=w2509, "New_State"=1, "State Machine in"=w2511) -> ("error out"=w2490:errorcluster, "State Machine out"=w2491:refnum<class "State Machine.lvclass">)  [unwired: 7 in]
              n933 = Increment(x=w2484) -> (x+1=w2483:u32)
              n934 = call-dynamic "Write Timer.vi"("error in (no error)"=w2490, "Timer"=u32 40, "State Machine in"=w2491) -> ("error out"=w2487:errorcluster, "State Machine out"=w2488:refnum<class "State Machine.lvclass">)  [unwired: 7 in]
              n935 = call-dynamic "Init Ticks2.vi"("error in (no error)"=w2487, "State Machine in"=w2488) -> ("error out"=w2486:errorcluster, "State Machine out"=w2485:refnum<class "State Machine.lvclass">)  [unwired: 8 in]
              n936 = call-dynamic "Write State Machine.vi"("error in (no error)"=w2486, "State Machine.lvclass"=w2485, "Device in"=w2508) -> ("error out"=w2492:errorcluster, "Device out"=w2494:refnum<class "Opt_Selector.lvclass">)  [unwired: 7 in]
            }
          }
          n937 = Bundle By Name(cluster=w2428, "seqAtual"=w2429) -> (w2427:refnum<class "S4GUI.lvclass">)
          n938 = call "Write WPROT.vi"("error in (no error)"=w2433, "Opt_Selector.lvclass"=w2435, "Instrument in"=w2434) -> ("error out"=w2437:errorcluster, "Instrument out"=w2436:refnum<class "Instrument.lvclass">)  [unwired: 7 in]
          n939 = call "Write Instrument.lvclass.vi"("error in (no error)"=w2437, "Instrument.lvclass"=w2436, "S4ACS_GUI in"=w2427) -> ("error out"=w2466:errorcluster, "S4ACS_GUI out"=w2465:refnum<class "S4GUI.lvclass">)  [unwired: 7 in]
          n940 = Bundle By Name(cluster=w2465, "Obs_state"=w2463) -> (w2462:refnum<class "S4GUI.lvclass">)
        }
        frame 304 {
          # "Espera terminar o movimento da lamina para disparar a aquisição\ndos canais ativos.\n\nOV 20230424: Não precisa mais atualizar o valor de WPPOS com o\ncomando WRITE_HEADER porque o ACS já recebeu a sequência de\nposições da lâmina."
          n941 = flat-sequence {
            tunnel: w2538 -> [w2563]
            tunnel: [w2563] -> w2537
            frame #0 {
              n942 = Tick Count (ms)() -> (millisecond timer value=w2562:u32)
              "time 2" <- w2562
              n943 = local read "time1"() -> (w2561:u32)
              n944 = Subtract(x=w2562, y=w2561) -> (x-y=→"delay wp":u32)
            }
          }
          n945 = call "Read Instrument.lvclass.vi"("error in (no error)"=w2537, "S4ACS_GUI in"=w2545) -> ("error out"=w2550:errorcluster, "Instrument.lvclass"=w2551:refnum<class "Instrument.lvclass">, "S4ACS_GUI out"=w2547:refnum<class "S4GUI.lvclass">)  [unwired: 7 in]
          n946 = call "Read WPROT.vi"("error in (no error)"=w2550, "Instrument in"=w2551) -> ("error out"=w2544:errorcluster, "Opt_Selector.lvclass"=w2543:refnum<class "Opt_Selector.lvclass">, "Instrument out"=w2549:refnum<class "Instrument.lvclass">)  [unwired: 7 in]
          n947 = call-dynamic "Read State Machine.vi"("error in (no error)"=w2544, "Device in"=w2543) -> ("error out"=w2518:errorcluster, "State Machine.lvclass"=w2521:refnum<class "State Machine.lvclass">, "Device out"=w2541:refnum<class "Opt_Selector.lvclass">)  [unwired: 7 in]
          n948 = call-dynamic "Verif Clock 2.vi"("error in (no error)"=w2518, "period (ms)"=u32 20000 ("period"), "State Machine in"=w2521) -> ("error out"=w2517:errorcluster, "time elapsed"=→"time elapsed":u32, "State Machine out"=w2520:refnum<class "State Machine.lvclass">)  [unwired: 6 in]
          n949 = call-dynamic "Read Timeout 2.vi"("error in (no error)"=w2517, "State Machine in"=w2520) -> ("error out"=w2516:errorcluster, "Timeout 2"=w2524:bool, "State Machine out"=w2519:refnum<class "State Machine.lvclass">)  [unwired: 7 in]
          n950 = call-dynamic "Read State.vi"("error in (no error)"=w2516, "State Machine in"=w2519) -> ("error out"=w2535:errorcluster, "State"=w2539:i32, "State Machine out"=w2536:refnum<class "State Machine.lvclass">)  [unwired: 7 in]
          n951 = Equal To 0?(x=w2539) -> (x = 0?=w2527:bool)
          n952 = call-dynamic "Write State Machine.vi"("error in (no error)"=w2535, "State Machine.lvclass"=w2536, "Device in"=w2541) -> ("error out"=w2540:errorcluster, "Device out"=w2542:refnum<class "Opt_Selector.lvclass">)  [unwired: 7 in]
          n953 = call "Write WPROT.vi"("error in (no error)"=w2540, "Opt_Selector.lvclass"=w2542, "Instrument in"=w2549) -> ("error out"=w2546:errorcluster, "Instrument out"=w2548:refnum<class "Instrument.lvclass">)  [unwired: 7 in]
          n954 = call "Write Instrument.lvclass.vi"("error in (no error)"=w2546, "Instrument.lvclass"=w2548, "S4ACS_GUI in"=w2547) -> ("error out"=w2526:errorcluster, "S4ACS_GUI out"=w2515:refnum<class "S4GUI.lvclass">)  [unwired: 7 in]
          n955 = case shown="True" w2524 {
            tunnel: w2523 -> [w2553 _]
            tunnel: [w2553 u32 1 ("Obs_state")] -> w2522
            tunnel: w2515 -> [w2552 w2557]
            tunnel: [w2552 w2556] -> w2514
            frame False {
            }
            frame True {
              n956 = Bundle By Name(cluster=w2557, "Error Msg"="ERROR: moving waveplate timeout  (S4GUI:HandleObservationSync.vi - state 302)") -> (w2556:refnum<class "S4GUI.lvclass">)
            }
          }
          n957 = Unbundle By Name(w2515) -> ("cyclesDone"=w2531:u32, "seqAtual"=w2530:u32)
          n958 = Decrement(x=w2530) -> (x-1=w2512:u32)
          n959 = Add(x=w2531, y=w2512) -> (x+y=w2529:u32)
          n960 = Equal To 0?(x=w2529) -> (x = 0?=w2532:bool)
          n961 = case shown="True" w2532 {
            tunnel: [u32 308 ("t") u32 308 ("t")] -> w2533
            frame False {
              (unwired) u32 310 ("t")
              # "Não é 1a seq:\nvai direto para\nenvio do trigger"
            }
            frame True {
              # "1a sequencia:\nenvia EXPOSE"
            }
          }
          n962 = Select(t=w2533, s=w2527, f=w2522) -> (s? t:f=w2534:u32)
          n963 = Bundle By Name(cluster=w2514, "Obs_state"=w2534) -> (w2528:refnum<class "S4GUI.lvclass">)
        }
        frame 308 {
          n964 = call-dynamic "Read AcquisitionA.vi"("error in (no error)"=w2626, "S4ACS_GUI in"=w2627) -> ("error out"=w2581:errorcluster, "Acquisition.lvclass"=w2582:refnum<class "Acquisition.lvclass">, "S4ACS_GUI out"=w2629:refnum<class "S4GUI.lvclass">)  [unwired: 7 in]
          n965 = call-dynamic "Read enabled.vi"("error in (no error)"=w2581, "Server in"=w2582) -> ("error out"=w2580:errorcluster, "enabled"=w2567:bool, "Server out"=w2583:refnum<class "Acquisition.lvclass">)  [unwired: 7 in]
          n966 = call "Read connection.vi"("error in (no error)"=w2580, "Server in"=w2583) -> ("error out"=w2606:errorcluster, "connection"=w2590:bool, "Server out"=w2607:refnum<class "Acquisition.lvclass">)  [unwired: 7 in]
          n967 = And(x=w2590, y=w2567) -> (x .and. y?=w2591:bool)
          n968 = case shown="True" w2591 {
            tunnel: w2607 -> [w2736 w2752]
            tunnel: w2606 -> [w2735 w2751]
            tunnel: [w2736 w2749] -> w2630
            tunnel: [w2735 w2748] -> w2628
            tunnel: [w2732 u32 0 ("New_State")] -> w2596
            tunnel: w2567 -> [w2731 _]
            frame False {
              n969 = Select(t=u32 1, s=w2731, f=u32 0) -> (s? t:f=w2732:u32)
            }
            frame True {
              n970 = call-dynamic "Read Channel.vi"("error in (no error)"=w2751, "Acquisition in"=w2752) -> ("error out"=w2744:errorcluster, "Channel.lvclass"=w2743:refnum<class "Channel.lvclass">, "Acquisition out"=w2750:refnum<class "Acquisition.lvclass">)  [unwired: 7 in]
              n971 = call-dynamic "Read State Machine.vi"("error in (no error)"=w2744, "Device in"=w2743) -> ("error out"=w2745:errorcluster, "State Machine.lvclass"=w2747:refnum<class "State Machine.lvclass">, "Device out"=w2741:refnum<class "Channel.lvclass">)  [unwired: 7 in]
              n972 = call "Next State.vi"("error in (no error)"=w2745, "New_State"=50, "State Machine in"=w2747) -> ("error out"=w2738:errorcluster, "State Machine out"=w2739:refnum<class "State Machine.lvclass">)  [unwired: 7 in]
              n973 = call-dynamic "Write State Machine.vi"("error in (no error)"=w2738, "State Machine.lvclass"=w2739, "Device in"=w2741) -> ("error out"=w2740:errorcluster, "Device out"=w2742:refnum<class "Channel.lvclass">)  [unwired: 7 in]
              n974 = call-dynamic "Write Channel.vi"("error in (no error)"=w2740, "Channel.lvclass"=w2742, "Acquisition in"=w2750) -> ("error out"=w2748:errorcluster, "Acquisition out"=w2749:refnum<class "Acquisition.lvclass">)  [unwired: 7 in]
            }
          }
          n975 = call-dynamic "Write AcquisitionA.vi"("error in (no error)"=w2628, "Acquisition.lvclass"=w2630, "S4ACS_GUI in"=w2629) -> ("error out"=w2623:errorcluster, "S4ACS_GUI out"=w2624:refnum<class "S4GUI.lvclass">)  [unwired: 7 in]
          n976 = call "Read AcquisitionB.vi"("error in (no error)"=w2623, "S4ACS_GUI in"=w2624) -> ("error out"=w2577:errorcluster, "Acquisition.lvclass"=w2579:refnum<class "Acquisition.lvclass">, "S4ACS_GUI out"=w2621:refnum<class "S4GUI.lvclass">)  [unwired: 7 in]
          n977 = call-dynamic "Read enabled.vi"("error in (no error)"=w2577, "Server in"=w2579) -> ("error out"=w2576:errorcluster, "enabled"=w2566:bool, "Server out"=w2578:refnum<class "Acquisition.lvclass">)  [unwired: 7 in]
          n978 = call "Read connection.vi"("error in (no error)"=w2576, "Server in"=w2578) -> ("error out"=w2604:errorcluster, "connection"=w2588:bool, "Server out"=w2605:refnum<class "Acquisition.lvclass">)  [unwired: 7 in]
          n979 = And(x=w2588, y=w2566) -> (x .and. y?=w2589:bool)
          n980 = case shown="True" w2589 {
            tunnel: w2605 -> [w2714 w2730]
            tunnel: w2604 -> [w2713 w2729]
            tunnel: [w2714 w2727] -> w2622
            tunnel: [w2713 w2726] -> w2620
            tunnel: [w2710 u32 0 ("New_State")] -> w2595
            tunnel: w2566 -> [w2709 _]
            frame False {
              n981 = Select(t=u32 2, s=w2709, f=u32 0) -> (s? t:f=w2710:u32)
            }
            frame True {
              n982 = call-dynamic "Read Channel.vi"("error in (no error)"=w2729, "Acquisition in"=w2730) -> ("error out"=w2722:errorcluster, "Channel.lvclass"=w2721:refnum<class "Channel.lvclass">, "Acquisition out"=w2728:refnum<class "Acquisition.lvclass">)  [unwired: 7 in]
              n983 = call-dynamic "Read State Machine.vi"("error in (no error)"=w2722, "Device in"=w2721) -> ("error out"=w2723:errorcluster, "State Machine.lvclass"=w2725:refnum<class "State Machine.lvclass">, "Device out"=w2719:refnum<class "Channel.lvclass">)  [unwired: 7 in]
              n984 = call "Next State.vi"("error in (no error)"=w2723, "New_State"=50, "State Machine in"=w2725) -> ("error out"=w2716:errorcluster, "State Machine out"=w2717:refnum<class "State Machine.lvclass">)  [unwired: 7 in]
              n985 = call-dynamic "Write State Machine.vi"("error in (no error)"=w2716, "State Machine.lvclass"=w2717, "Device in"=w2719) -> ("error out"=w2718:errorcluster, "Device out"=w2720:refnum<class "Channel.lvclass">)  [unwired: 7 in]
              n986 = call-dynamic "Write Channel.vi"("error in (no error)"=w2718, "Channel.lvclass"=w2720, "Acquisition in"=w2728) -> ("error out"=w2726:errorcluster, "Acquisition out"=w2727:refnum<class "Acquisition.lvclass">)  [unwired: 7 in]
            }
          }
          n987 = call "Write AcquisitionB.vi"("error in (no error)"=w2620, "Acquisition.lvclass"=w2622, "S4ACS_GUI in"=w2621) -> ("error out"=w2616:errorcluster, "S4ACS_GUI out"=w2615:refnum<class "S4GUI.lvclass">)  [unwired: 7 in]
          n988 = call-dynamic "Read AcquisitionC.vi"("error in (no error)"=w2616, "S4ACS_GUI in"=w2615) -> ("error out"=w2573:errorcluster, "Acquisition.lvclass"=w2575:refnum<class "Acquisition.lvclass">, "S4ACS_GUI out"=w2618:refnum<class "S4GUI.lvclass">)  [unwired: 7 in]
          n989 = call-dynamic "Read enabled.vi"("error in (no error)"=w2573, "Server in"=w2575) -> ("error out"=w2572:errorcluster, "enabled"=w2565:bool, "Server out"=w2574:refnum<class "Acquisition.lvclass">)  [unwired: 7 in]
          n990 = call "Read connection.vi"("error in (no error)"=w2572, "Server in"=w2574) -> ("error out"=w2602:errorcluster, "connection"=w2585:bool, "Server out"=w2603:refnum<class "Acquisition.lvclass">)  [unwired: 7 in]
          n991 = And(x=w2585, y=w2565) -> (x .and. y?=w2587:bool)
          n992 = case shown="True" w2587 {
            tunnel: [w2691 w2700] -> w2619
            tunnel: [w2692 w2699] -> w2617
            tunnel: w2603 -> [w2692 w2697]
            tunnel: w2602 -> [w2691 w2696]
            tunnel: [w2688 u32 0 ("New_State")] -> w2594
            tunnel: w2565 -> [w2687 _]
            frame False {
              n993 = Select(t=u32 4, s=w2687, f=u32 0) -> (s? t:f=w2688:u32)
            }
            frame True {
              n994 = call-dynamic "Read Channel.vi"("error in (no error)"=w2696, "Acquisition in"=w2697) -> ("error out"=w2704:errorcluster, "Channel.lvclass"=w2705:refnum<class "Channel.lvclass">, "Acquisition out"=w2698:refnum<class "Acquisition.lvclass">)  [unwired: 7 in]
              n995 = call-dynamic "Read State Machine.vi"("error in (no error)"=w2704, "Device in"=w2705) -> ("error out"=w2703:errorcluster, "State Machine.lvclass"=w2701:refnum<class "State Machine.lvclass">, "Device out"=w2707:refnum<class "Channel.lvclass">)  [unwired: 7 in]
              n996 = call "Next State.vi"("error in (no error)"=w2703, "New_State"=50, "State Machine in"=w2701) -> ("error out"=w2695:errorcluster, "State Machine out"=w2694:refnum<class "State Machine.lvclass">)  [unwired: 7 in]
              n997 = call-dynamic "Write State Machine.vi"("error in (no error)"=w2695, "State Machine.lvclass"=w2694, "Device in"=w2707) -> ("error out"=w2708:errorcluster, "Device out"=w2706:refnum<class "Channel.lvclass">)  [unwired: 7 in]
              n998 = call-dynamic "Write Channel.vi"("error in (no error)"=w2708, "Channel.lvclass"=w2706, "Acquisition in"=w2698) -> ("error out"=w2700:errorcluster, "Acquisition out"=w2699:refnum<class "Acquisition.lvclass">)  [unwired: 7 in]
            }
          }
          n999 = call-dynamic "Write AcquisitionC.vi"("error in (no error)"=w2619, "Acquisition.lvclass"=w2617, "S4ACS_GUI in"=w2618) -> ("error out"=w2613:errorcluster, "S4ACS_GUI out"=w2612:refnum<class "S4GUI.lvclass">)  [unwired: 7 in]
          n1000 = call-dynamic "Read AcquisitionD.vi"("error in (no error)"=w2613, "S4ACS_GUI in"=w2612) -> ("error out"=w2569:errorcluster, "Acquisition.lvclass"=w2571:refnum<class "Acquisition.lvclass">, "S4ACS_GUI out"=w2611:refnum<class "S4GUI.lvclass">)  [unwired: 7 in]
          n1001 = call-dynamic "Read enabled.vi"("error in (no error)"=w2569, "Server in"=w2571) -> ("error out"=w2568:errorcluster, "enabled"=w2564:bool, "Server out"=w2570:refnum<class "Acquisition.lvclass">)  [unwired: 7 in]
          n1002 = call "Read connection.vi"("error in (no error)"=w2568, "Server in"=w2570) -> ("error out"=w2600:errorcluster, "connection"=w2584:bool, "Server out"=w2601:refnum<class "Acquisition.lvclass">)  [unwired: 7 in]
          n1003 = And(x=w2584, y=w2564) -> (x .and. y?=w2586:bool)
          n1004 = case shown="True" w2586 {
            tunnel: w2600 -> [w2669 w2686]
            tunnel: [w2669 w2685] -> w2614
            tunnel: w2601 -> [w2670 w2676]
            tunnel: [w2670 w2674] -> w2610
            tunnel: [w2666 u32 0 ("New_State")] -> w2593
            tunnel: w2564 -> [w2665 _]
            frame False {
              n1005 = Select(t=u32 8, s=w2665, f=u32 0) -> (s? t:f=w2666:u32)
            }
            frame True {
              n1006 = call-dynamic "Read Channel.vi"("error in (no error)"=w2686, "Acquisition in"=w2676) -> ("error out"=w2681:errorcluster, "Channel.lvclass"=w2680:refnum<class "Channel.lvclass">, "Acquisition out"=w2675:refnum<class "Acquisition.lvclass">)  [unwired: 7 in]
              n1007 = call-dynamic "Read State Machine.vi"("error in (no error)"=w2681, "Device in"=w2680) -> ("error out"=w2682:errorcluster, "State Machine.lvclass"=w2684:refnum<class "State Machine.lvclass">, "Device out"=w2678:refnum<class "Channel.lvclass">)  [unwired: 7 in]
              n1008 = call "Next State.vi"("error in (no error)"=w2682, "New_State"=50, "State Machine in"=w2684) -> ("error out"=w2672:errorcluster, "State Machine out"=w2673:refnum<class "State Machine.lvclass">)  [unwired: 7 in]
              n1009 = call-dynamic "Write State Machine.vi"("error in (no error)"=w2672, "State Machine.lvclass"=w2673, "Device in"=w2678) -> ("error out"=w2677:errorcluster, "Device out"=w2679:refnum<class "Channel.lvclass">)  [unwired: 7 in]
              n1010 = call-dynamic "Write Channel.vi"("error in (no error)"=w2677, "Channel.lvclass"=w2679, "Acquisition in"=w2675) -> ("error out"=w2685:errorcluster, "Acquisition out"=w2674:refnum<class "Acquisition.lvclass">)  [unwired: 7 in]
            }
          }
          n1011 = call-dynamic "Write AcquisitionD.vi"("error in (no error)"=w2614, "Acquisition.lvclass"=w2610, "S4ACS_GUI in"=w2611) -> ("error out"=w2609:errorcluster, "S4ACS_GUI out"=w2608:refnum<class "S4GUI.lvclass">)  [unwired: 7 in]
          n1012 = Compound Arithmetic op=ADD(w2596, w2595, w2594, w2593) -> (w2597:u32)
          n1013 = case shown="2" w2597 {
            tunnel: w2592 -> [w2634 _ _ _ _ _ _ _ _ _ _ _ _ _ _ _]
            tunnel: [w2633 u32 1 ("Obs_state") u32 1 ("Obs_state") u32 1 ("Obs_state") u32 1 ("Obs_state") u32 1 ("Obs_state") u32 1 ("Obs_state") u32 1 ("Obs_state") u32 1 ("Obs_state") u32 1 ("Obs_state") u32 1 ("Obs_state") u32 1 ("Obs_state") u32 1 ("Obs_state") u32 1 ("Obs_state") u32 1 ("Obs_state") u32 1 ("Obs_state")] -> w2598
